vi "Base64 Encode.vi"(8 "error in (no error)":errorcluster, 11 "string in (not encoded)":string) -> (0 "error out":errorcluster, 3 "string out (base64-encoded)":string)   [LabVIEW 2026]
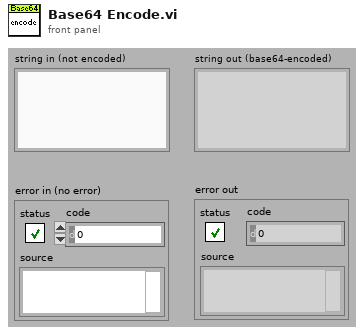
[diagram p1: front panel]
types:
  T1 = cluster{"unsigned byte array[0]":u8, "unsigned byte array[1]":u8, "unsigned byte array[2]":u8}
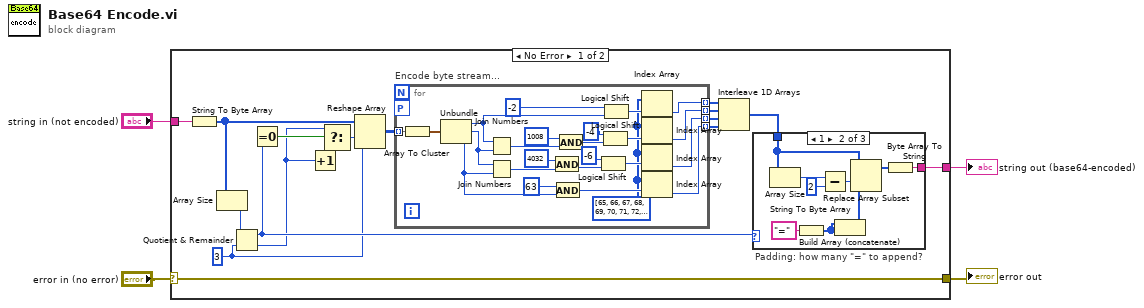
[diagram p0: block diagram]
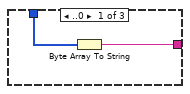
[diagram p2: hidden frame]
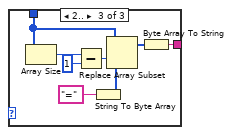
[diagram p3: hidden frame]
diagram:
  n1 = case shown="No Error" "error in (no error)" {
    selector: "error in (no error)" -> [w21 w66]
    tunnel: "string in (not encoded)" -> [w6 w65]
    tunnel: [w21 w66] -> w2
    tunnel: [w5 w65] -> w1
    frame No Error {
      w9 = 3 ("y")
      n2 = String To Byte Array(string=w6) -> (unsigned byte array=w10:u8[])
      n3 = Array Size(array=w10) -> (size(s)=w18:i32)
      n4 = Quotient & Remainder(x=w18, y=w9) -> (x-y*floor(x/y)=w19:i32, floor(x/y)=w12:i32)
      n5 = Equal To 0?(x=w19) -> (x = 0?=w20:bool)
      n6 = Increment(x=w12) -> (x+1=w13:i32)
      n7 = Select(t=w12, s=w20, f=w13) -> (s? t:f=w8:i32)
      n8 = Reshape Array(w10, w8, w9) -> (w7:u8[][])
      n9 = for "Encode byte stream..." {
        tunnel: [w24] -> w14 mode=indexing
        tunnel: [w25] -> w15 mode=indexing
        tunnel: [w26] -> w16 mode=indexing
        tunnel: [w27] -> w17 mode=indexing
        workers-P: _ -> [_]
        tunnel: w7 -> [w22] mode=indexing
        w23 = u8[] [65, 66, 67, 68, 69, 70, 71, 72, 73, 74, 75, 76, 77, 78, 79, 80, 81, 82, 83, 84, 85, 86, 87, 88, 89, 90, 97, 98, 99, 100, 101, 102, 103, 104, 105, 106, 107, 108, 109, 110, 111, 112, 113, 114, 115, 116, 117, 118, 119, 120, 121, 122, 48, 49, 50, 51, 52, 53, 54, 55, 56, 57, 43, 47] ("unsigned byte array")
        n10 = Array To Cluster(array=w22) -> (cluster=w45:T1)
        n11 = Unbundle(w45) -> ("unsigned byte array[0]"=w34:u8, "unsigned byte array[1]"=w39:u8, "unsigned byte array[2]"=w33:u8)
        n12 = Join Numbers(hi=w34, lo=w39) -> ((hi.lo)=w43:u16)
        n13 = Join Numbers(hi=w39, lo=w33) -> ((hi.lo)=w38:u16)
        n14 = And(x=u16 4032, y=w38) -> (x .and. y?=w36:u16)
        n15 = And(x=u8 63, y=w33) -> (x .and. y?=w28:u8)
        n16 = And(x=u16 1008, y=w43) -> (x .and. y?=w41:u16)
        n17 = Logical Shift(y=i8 -6, x=w36) -> (x << y=w29:u16)
        n18 = Logical Shift(y=i8 -4, x=w41) -> (x << y=w30:u16)
        n19 = Logical Shift(y=i8 -2, x=w34) -> (x << y=w31:u8)
        n20 = Index Array(array=w23, index=w31) -> (element=w27:u8)
        n21 = Index Array(array=w23, index=w30) -> (element=w26:u8)
        n22 = Index Array(array=w23, index=w29) -> (element=w25:u8)
        n23 = Index Array(array=w23, index=w28) -> (element=w24:u8)
      }
      n24 = Interleave 1D Arrays(w17, w16, w15, w14) -> (w11:u8[])
      n25 = case "Padding: how many \"=\" to append?" shown="1" w19 {
        tunnel: [w46 w53 w61] -> w5
        tunnel: w11 -> [w47 w51 w59]
        frame ..0 {
          n26 = Byte Array To String(unsigned byte array=w47) -> (string=w46:string)
        }
        frame 1 {
          n27 = Array Size(array=w51) -> (size(s)=w52:i32)
          n28 = String To Byte Array(string="=") -> (unsigned byte array=w49:u8[])
          n29 = Subtract(x=w52, y=2) -> (x-y=w55:i32)
          n30 = Build Array (concatenate)(w49, w49) -> (w48:u8[])
          n31 = Replace Array Subset(array=w51, new element=w48, index=w55) -> (w54:u8[])
          n32 = Byte Array To String(unsigned byte array=w54) -> (string=w53:string)
        }
        frame 2.. {
          n33 = Array Size(array=w59) -> (size(s)=w60:i32)
          n34 = Subtract(x=w60, y=1) -> (x-y=w63:i32)
          n35 = String To Byte Array(string="=") -> (unsigned byte array=w57:u8[])
          n36 = Replace Array Subset(array=w59, new element=w57, index=w63) -> (w62:u8[])
          n37 = Byte Array To String(unsigned byte array=w62) -> (string=w61:string)
        }
      }
    }
    frame Error {
    }
  }
  "string out (base64-encoded)" <- w1
  "error out" <- w2
